vi "SVErrorSource.vi"(6 "RT?":bool, 8 "error in":errorcluster, 9 "Resolved URL":string, 10 "Unresolved URL":string, 11 "Write?":bool) -> (0 "error out":errorcluster)   [LabVIEW 2017]
panel:
  in  "Error":string="error"
  in  "Warning":string="warning"
  in  "Format String":string="Shared Variable %s in %s\n<append>\nThis %s occurred while %s %s (%s)"
  in  "reading":string="reading"
  in  "writing":string="writing"
  in  "Read":string="Read"
  in  "Write":string="Write"
  # "L10N"
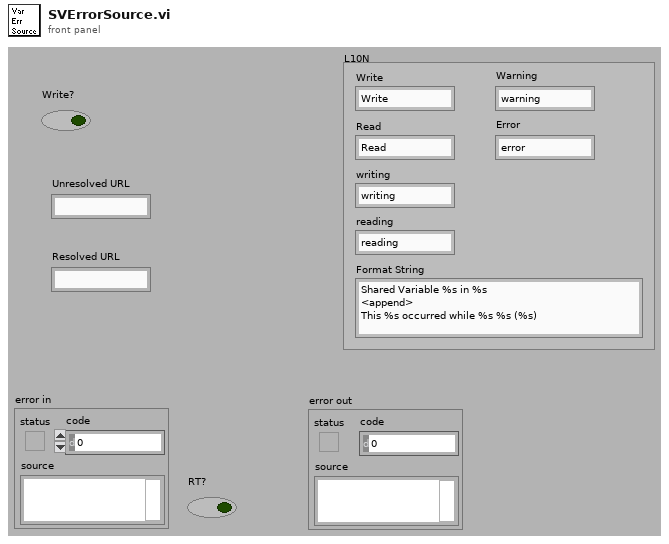
[diagram p1: front panel]
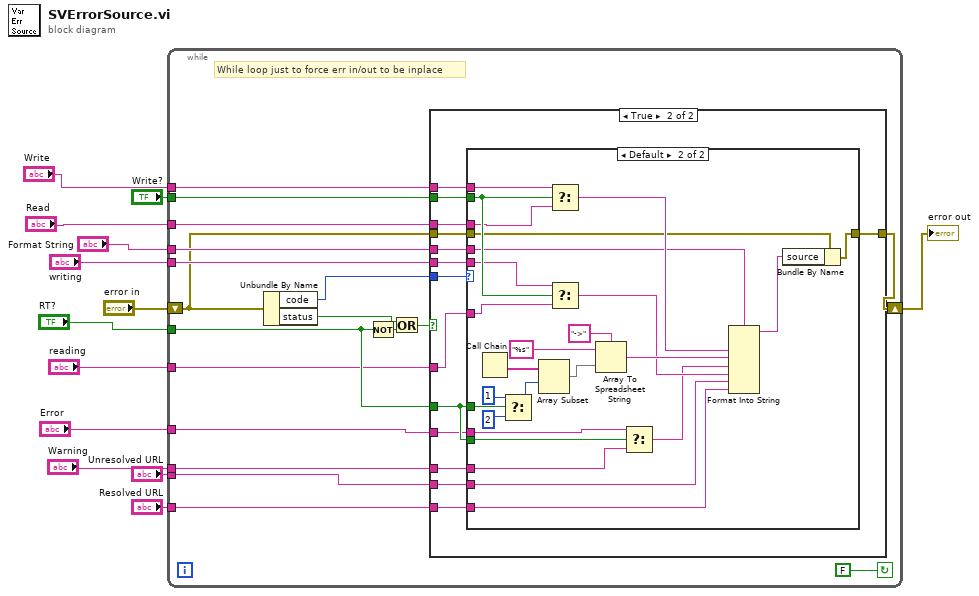
[diagram p0: block diagram]
diagram:
  n1 = while {
    tunnel: "Write?" -> [w31]
    tunnel: "Unresolved URL" -> [w30]
    tunnel: "Resolved URL" -> [w29]
    tunnel: "RT?" -> [w26]
    tunnel: "Write" -> [w24]
    tunnel: "Read" -> [w23]
    tunnel: "writing" -> [w22]
    tunnel: "reading" -> [w21]
    tunnel: "Error" -> [w20]
    tunnel: "Warning" -> [w19]
    tunnel: "Format String" -> [w18]
    shift-right: [w28] -> w10
    shift-left: "error in" -> [w14]
    stop <- FALSE continue-if-true
    # "While loop just to force err in/out to be inplace"
    n2 = Unbundle By Name(w14) -> ("code"=w17:i32, "status"=w16:bool)
    n3 = Not(x=w26) -> (.not. x?=w25:bool)
    n4 = Or(x=w16, y=w25) -> (x .or. y?=w27:bool)
    n5 = case shown="True" w27 {
      tunnel: w31 -> [_ w46]
      tunnel: w30 -> [_ w45]
      tunnel: w29 -> [_ w44]
      tunnel: [w32 w43] -> w28
      tunnel: w14 -> [w32 w33]
      tunnel: w17 -> [_ w42]
      tunnel: w26 -> [_ w41]
      tunnel: w24 -> [_ w40]
      tunnel: w23 -> [_ w39]
      tunnel: w22 -> [_ w38]
      tunnel: w21 -> [_ w37]
      tunnel: w20 -> [_ w36]
      tunnel: w19 -> [_ w35]
      tunnel: w18 -> [_ w34]
      frame False {
      }
      frame True {
        n6 = case shown="Default" w42 {
          tunnel: w46 -> [_ w65]
          tunnel: w45 -> [_ w66]
          tunnel: w44 -> [_ w67]
          tunnel: [w47 w49] -> w43
          tunnel: w41 -> [_ w62]
          tunnel: w41 -> [_ w60]
          tunnel: w40 -> [_ w57]
          tunnel: w39 -> [_ w56]
          tunnel: w38 -> [_ w55]
          tunnel: w37 -> [_ w54]
          tunnel: w36 -> [_ w53]
          tunnel: w35 -> [_ w52]
          tunnel: w34 -> [_ w51]
          tunnel: w33 -> [w47 w48]
          frame 0 {
          }
          frame Default {
            n7 = Call Chain() -> (call chain=w69:string[])
            n8 = Select(t=1 ("index"), s=w60, f=2 ("index")) -> (s? t:f=w61:i32)
            n9 = Array Subset(array=w69, index=w61) -> (w68:string[])  [unwired: 1 in]
            n10 = Select(t=w57, s=w65, f=w56) -> (s? t:f=w72:string)
            n11 = Select(t=w55, s=w65, f=w54) -> (s? t:f=w59:string)
            n12 = Array To Spreadsheet String(delimiter (Tab)="->", array=w68, 3:"%s" ("format string")) -> (spreadsheet string=w71:string)
            n13 = Select(t=w53, s=w62, f=w52) -> (s? t:f=w58:string)
            n14 = Format Into String(format string=w51, w72, w71, w58, w59, w66, w67) -> (resulting string=w50:string)  [unwired: 2 in, 1 out]
            n15 = Bundle By Name(cluster=w48, "source"=w50) -> (w49:errorcluster)
          }
        }
      }
    }
  }
  "error out" <- w10
